vi "User Access Level FGV.vi"(7 "用户等级命令":T1, 8 "错误输入":cluster{"状态":bool, "代码":i32, "源":string}, 10 "用户名":string) -> (0 "错误输出":cluster{"状态":bool, "代码":i32, "源":string}, 1 "用户级别":string)   [LabVIEW 2012]
doc: "该FGV中保存了当前登录用户的访问级别，可执行以下方法：\n\n1. <B>读取用户访问级别文件：</B> 读取一个制表符分隔的文本文件，其中包含用户命和相应的访问级别。\n2. <B>设置当前访问级别：</B> 为输入的用户名设置访问级别。\n3. <B>获取当前访问级别：</B> 返回当前用户的访问级别。"
uses:
  User Access Level Method.ctl
  <vilib>/Utility/file.llb/Read From Spreadsheet File (string).vi
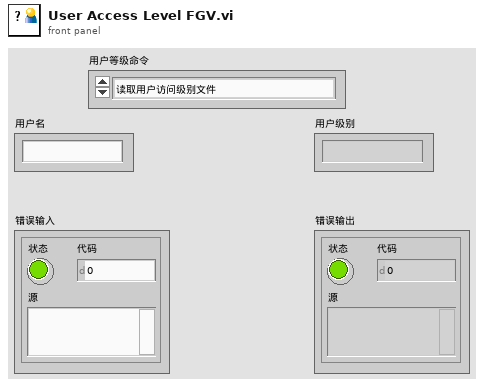
[diagram p1: front panel]
types:
  T1 = typedef "User Access Level Method.ctl" = enum16{"读取用户访问级别文件", "设置当前访问级别", "获取当前访问级别"}
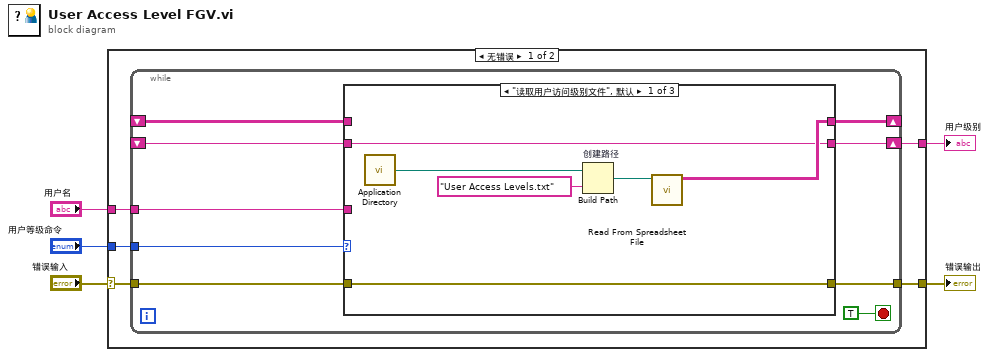
[diagram p0: block diagram]
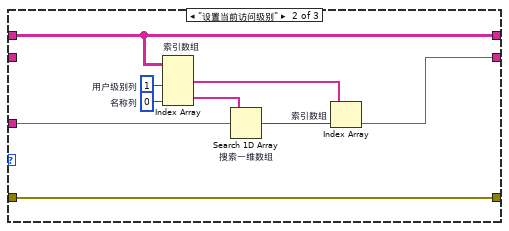
[diagram p2: hidden frame]
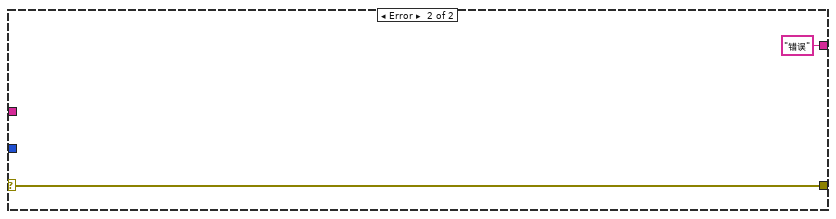
[diagram p4: hidden frame]
diagram:
  n1 = case shown="无错误" "错误输入" {
    selector: "错误输入" -> [w6 w39]
    tunnel: "用户等级命令" -> [w10 _]
    tunnel: [w9 w39] -> w4
    tunnel: "用户名" -> [w8 _]
    tunnel: [w7 "错误" ("字符串")] -> w2
    frame No Error {
      n2 = while {
        tunnel: w10 -> [w18]
        tunnel: [w17] -> w9
        tunnel: w6 -> [w16]
        shift-right: [w15] -> _
        shift-left: _ -> [w14]
        tunnel: w8 -> [w13]
        shift-right: [w12] -> w7
        shift-left: _ -> [w11]
        stop <- TRUE stop-if-true
        n3 = case shown="\"读取用户访问级别文件\", 默认" w18 {
          tunnel: [w25 w34 w37] -> w17
          tunnel: w16 -> [w25 w34 w37]
          tunnel: [w22 w33 w36] -> w15
          tunnel: w14 -> [_ w33 w36]
          tunnel: w13 -> [_ w31 _]
          tunnel: [w21 w27 w35] -> w12
          tunnel: w11 -> [w21 _ w35]
          frame "读取用户访问级别文件", Default {
            n4 = call <vilib>:"Application Directory.vi"() -> ("Application Directory"=w20:path)
            n5 = Build Path "创建路径"(base path=w20, name or relative path="User Access Levels.txt" ("名称或相对路径")) -> (appended path=w23:path)
            n6 = call-poly <vilib>:"Read From Spreadsheet File.vi"("file path (dialog if empty)"=w23) -> ("all rows"=w22:string[][])  [unwired: 6 in, 4 out]
          }
          frame "设置当前访问级别" {
            w30 = 1  # 用户级别列
            w32 = 0  # 名称列
            n7 = Index Array "索引数组"(array=w33, index (col) #1=w30, index (col) #2=w32) -> (element #1=w28:string[], element #2=w26:string[])  [unwired: 2 in]
            n8 = Search 1D Array "搜索一维数组"(1D array=w26, element=w31) -> (index of element=w29:i32)  [unwired: 1 in]
            n9 = Index Array "索引数组"(array=w28, index=w29) -> (element=w27:string)
          }
          frame "获取当前访问级别" {
          }
        }
      }
    }
    frame Error {
    }
  }
  "用户级别" <- w2
  "错误输出" <- w4
